vi "Aerotech Dumbness Fixer.vi"   [LabVIEW 2017]
panel:
  # "Run this VI.\n\nWhen it's finished, select \"Quit.\" then \"Save\"\n\nLabVIEW will restart.\n\nAerotech Drivers will be available in\nthe Functions Pallete @ \nUser Libraries>>aerotech\n\nAfter LabVIEW restarts move\n\nC:\\Program Files\\Aerotech\\LabVIEW\\8.2\nto\nC:\\Program Files\\Aerotech\\LabVIEW\\8.2\\DoNotUse\nThis should prevent conflicts.\n\nShazam."
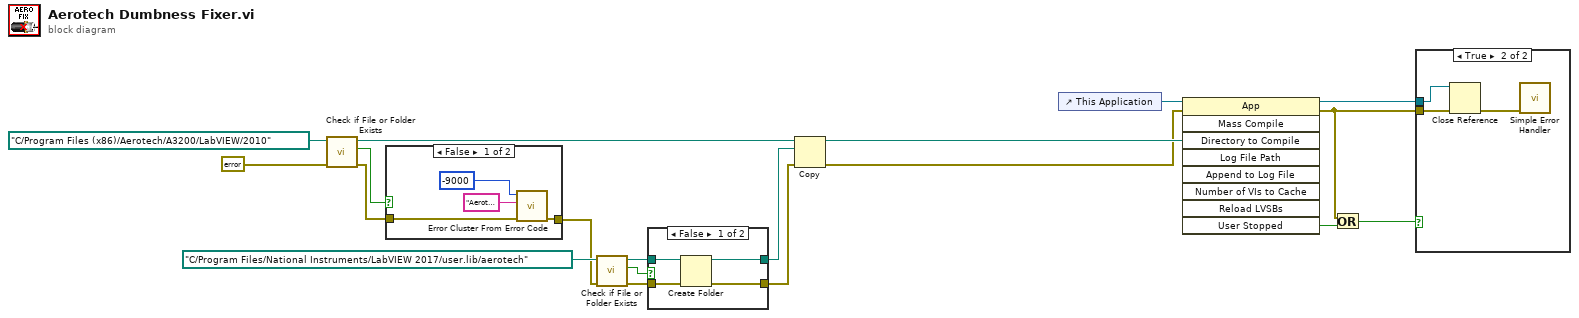
[diagram p0: block diagram]
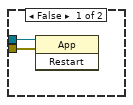
[diagram p2: hidden frame]
diagram:
  n1 = call <vilib>:"Check if File or Folder Exists.vi"("error in (no error)"=errorcluster {"status"=FALSE, "code"=0, "source"=""} ("error constant"), "path"=path "C:/Program Files (x86)/Aerotech/A3200/LabVIEW/2010") -> ("error out"=w10:errorcluster, "file or folder exists?"=w11:bool, "dup path"=w2:path)  [unwired: 7 in]
  n2 = case shown="False" w11 {
    tunnel: w10 -> [w23 w24]
    tunnel: [w20 w24] -> w9
    frame False {
      n3 = call <vilib>:"Error Cluster From Error Code.vi"("error in (no error)"=w23, "error message (\"\")"="Aerotech drivers are not installed at the expected location." ("error message (\"\")"), "error code (0)"=-9000) -> ("error out"=w20:errorcluster)  [unwired: 6 in]
    }
    frame True {
    }
  }
  n4 = call <vilib>:"Check if File or Folder Exists.vi"("error in (no error)"=w9, "path"=path "C:/Program Files/National Instruments/LabVIEW 2017/user.lib/aerotech" ("target path (use dialog)")) -> ("error out"=w15:errorcluster, "file or folder exists?"=w17:bool, "dup path"=w16:path)  [unwired: 7 in]
  n5 = case shown="False" w17 {
    tunnel: w16 -> [w28 w30]
    tunnel: w15 -> [w27 w29]
    tunnel: [w26 w30] -> w14
    tunnel: [w25 w29] -> w13
    frame False {
      n6 = Create Folder(path (use dialog)=w28, error in=w27) -> (created path=w26:path, error out=w25:errorcluster)  [unwired: 1 in, 1 out]
    }
    frame True {
    }
  }
  n7 = Copy(8:w13, 10:w14, 11:w2) -> (0:w1:errorcluster, 3:w7:path)  [unwired: 2 in, 1 out]
  n8 = control-ref of="This Application"() -> (w8:refnum<vi>)
  n9 = invoke class="App" method="Mass Compile"(reference=w8, error in=w1, "Directory to Compile"=w7) -> (reference out=w3:refnum<vi>, error out=w4:errorcluster, "User Stopped"=w5:bool)  [unwired: 6 in, 6 out]
  n10 = Or(x=w4, y=w5) -> (x .or. y?=w6:bool)
  n11 = case shown="True" w6 {
    tunnel: w4 -> [w32 w34]
    tunnel: w3 -> [w31 w35]
    frame False {
      n12 = invoke class="App" method="Restart"(reference=w31, error in=w32) -> ()  [unwired: 1 in, 3 out]
    }
    frame True {
      n13 = Close Reference(reference=w35, error in (no error)=w34) -> (error out=w33:errorcluster)
      n14 = call <vilib>:"Simple Error Handler.vi"("error in (no error)"=w33) -> ()  [unwired: 4 in, 5 out]
    }
  }
